vi "MainIdent RT.vi"   [LabVIEW 2018]
doc: "The myRIO Project template acquires acceleration data from the onboard accelerometer and displays the changes of acceleration values in a waveform chart."
uses:
  <vilib>/myRIO/Common/Instrument Driver Framework/myRIO v1.0/Encoder/typedefs/Encoder Signal Mode.ctl
  <vilib>/Platform/TimedLoop/XDataNode/timing_clust.ctl
  <vilib>/Platform/TimedLoop/XDataNode/nitl_modes.ctl
  <vilib>/Platform/TimedLoop/XDataNode/wakeup.ctl
  <vilib>/myRIO/Instrument Drivers/Onboard IO/PWM/typedefs/PWM Reference.ctl
  <vilib>/myRIO/Common/Instrument Driver Framework/Utilities/typedefs/myRIO Generic Hardware Reference.ctl
  <vilib>/myRIO/Common/Instrument Driver Framework/Utilities/typedefs/Hardware Version Enum.ctl
  <vilib>/myRIO/Common/Instrument Driver Framework/Utilities/typedefs/myRIO v1.0 Reference.ctl
  <vilib>/myRIO/Common/Instrument Driver Framework/Utilities/typedefs/Generic FPGA Reference.ctl
  <vilib>/myRIO/Common/Instrument Driver Framework/myRIO v1.0/PWM/typedefs/PWM Channels Enum.ctl
  <vilib>/myRIO/Instrument Drivers/Onboard IO/PWM/typedefs/PWM Configuration.ctl
  <vilib>/userdefined/High Color/nirio_resource_hc.ctl
  <vilib>/myRIO/Common/Instrument Driver Framework/myRIO v1.0/Encoder/typedefs/Encoder Configuration v1.0.ctl
  <vilib>/myRIO/Instrument Drivers/Onboard IO/Encoder/typedefs/Encoder Reference.ctl
  <vilib>/myRIO/Common/Instrument Driver Framework/myRIO v1.0/Encoder/typedefs/Encoder Channels Enum.ctl
  <vilib>/myRIO/Common/Instrument Driver Framework/myRIO v1.0/PWM/vis/myRIO v1.1 Open PWM.vi
  <vilib>/myRIO/Common/Instrument Driver Framework/myRIO v1.0/Encoder/vis/myRIO v1.1 Open Encoder.vi
  <vilib>/myRIO/Common/Instrument Driver Framework/Utilities/vis/Validate Channels.vi
  <vilib>/myRIO/Common/Instrument Driver Framework/myRIO v1.0/PWM/vis/myRIO v1.0 Reserve PWM.vi
  <vilib>/myRIO/Instrument Drivers/Onboard IO/PWM/vis/Set Duty Cycle and Frequency.vi
  <vilib>/myRIO/Common/Instrument Driver Framework/myRIO v1.0/Encoder/vis/myRIO v1.0 Reserve Encoder.vi
  <vilib>/myRIO/Common/Instrument Driver Framework/myRIO v1.0/Encoder/vis/myRIO v1.0 Close Encoder.vi
  <vilib>/myRIO/Common/Instrument Driver Framework/myRIO v1.0/PWM/vis/myRIO v1.0 Close PWM.vi
  <vilib>/myRIO/Common/Instrument Driver Framework/myRIO v1.0/PWM/vis/myRIO v1.0 Build MUX Configuration PWM.vi
  <vilib>/myRIO/Common/Instrument Driver Framework/myRIO v1.0/Resource Manager/vis/myRIO v1.0 Reserve Channel List.vi
  <vilib>/myRIO/Common/Instrument Driver Framework/myRIO v1.0/Encoder/vis/myRIO v1.0 Build MUX Configuration Encoder.vi
  <vilib>/myRIO/Common/Instrument Driver Framework/myRIO v1.0/Encoder/vis/myRIO v1.0 Unreserve Encoder.vi
  <vilib>/myRIO/Common/Instrument Driver Framework/myRIO v1.0/PWM/vis/myRIO v1.0 Unreserve PWM.vi
  <vilib>/myRIO/Common/Instrument Driver Framework/myRIO v1.0/Resource Manager/vis/myRIO v1.0 Create Configuration List.vi
  <vilib>/myRIO/Common/Instrument Driver Framework/myRIO v1.0/Resource Manager/vis/myRIO v1.0 Reserve Channel.vi
  <vilib>/myRIO/Common/Instrument Driver Framework/myRIO v1.0/Resource Manager/vis/myRIO v1.0 Unreserve Channel.vi
  <vilib>/myRIO/Common/Instrument Driver Framework/myRIO v1.0/Resource Manager/vis/myRIO v1.0 Unreserve Channel List.vi
  <vilib>/myRIO/Common/Instrument Driver Framework/myRIO v1.0/Resource Manager/vis/myRIO v1.0 Build Mutex Name.vi
  <vilib>/Utility/VariantDataType/GetNumericInfo.vi
  <vilib>/Utility/error.llb/Error Cluster From Error Code.vi
  <vilib>/myRIO/Common/Instrument Driver Framework/myRIO v1.0/myRIO v1.1 Open.vi
  <vilib>/myRIO/Common/Instrument Driver Framework/Utilities/vis/IO Manager.vi
  <vilib>/myRIO/Common/Instrument Driver Framework/Utilities/vis/Configuration Manager.vi
  <vilib>/myRIO/Common/Instrument Driver Framework/myRIO v1.0/Resource Manager/vis/myRIO v1.0 Configure IO.vi
  <vilib>/myRIO/Common/Instrument Driver Framework/myRIO v1.0/myRIO v1.0 Close.vi
  <vilib>/myRIO/Common/Instrument Driver Framework/myRIO v1.0/PWM/vis/myRIO v1.0 Write PWM.vi
  <vilib>/myRIO/Common/Instrument Driver Framework/myRIO v1.0/Encoder/vis/myRIO v1.0 Configure Encoder.vi
  <vilib>/myRIO/Common/Instrument Driver Framework/myRIO v1.0/Encoder/vis/myRIO v1.0 Enable Encoder.vi
  <vilib>/myRIO/Common/Instrument Driver Framework/myRIO v1.0/Encoder/vis/myRIO v1.0 Read Encoder.vi
  <vilib>/myRIO/Common/Instrument Driver Framework/myRIO v1.0/Encoder/vis/myRIO v1.0 Shutdown Encoder.vi
  <vilib>/myRIO/Common/Instrument Driver Framework/myRIO v1.0/PWM/vis/myRIO v1.0 Shutdown PWM.vi
  <vilib>/platform/TimedLoop/XDataNode/XDataNode.xnode
  <vilib>/myRIO/Instrument Drivers/Onboard IO/PWM/vis/myRIO PWM Open.xnode
  <vilib>/myRIO/Instrument Drivers/Onboard IO/Encoder/vis/myRIO Encoder Open.xnode
  <vilib>/Platform/TimedLoop/XDataNode/XDNodeRunTimeDep.lvlib
  <vilib>/myRIO/Instrument Drivers/Onboard IO/Encoder/Encoder.lvlib
  <vilib>/myRIO/Instrument Drivers/Onboard IO/PWM/PWM.lvlib
types:
  T1 = typedef "Encoder Signal Mode.ctl" = enum16{"Quadrature phase signal", "Step and direction signal"}
  T2 = typedef "PWM.lvlib/PWM Reference.ctl" = cluster{"myRIO Reference":T3, "PWM Channels Enum":T7, "PWM Configuration":T8}
  T3 = typedef "myRIO Generic Hardware Reference.ctl" = cluster{"myRIO Model":T4, "myRIO Hardware Reference":T5}
  T4 = typedef "Hardware Version Enum.ctl" = enum16{"Unknown", "myRIO-1900", "myRIO-1950", "roboRIO", "NI ELVIS RIO CM", "ELVIS III"}
  T5 = typedef "myRIO v1.0 Reference.ctl" = cluster{"Generic FPGA Reference":T6, "Allow multiple opens":bool}
  T6 = typedef "Generic FPGA Reference.ctl" = refnum<k20>
  T7 = typedef "PWM Channels Enum.ctl" = enum16{"Not Connected", "C/PWM0", "C/PWM1", "A/PWM0", "A/PWM1", "A/PWM2", "A/PWM3", "A/PWM4", "A/PWM5", "A/PWM6", "A/PWM7", "A/PWM8", "A/PWM9", "A/PWM10", "A/PWM11", "A/PWM12", "A/PWM13", "A/PWM14", "A/PWM15", "A/PWM16", "A/PWM17", "A/PWM18", "A/PWM19", "B/PWM0", "B/PWM1", "B/PWM2", "B/PWM3", "B/PWM4", "B/PWM5", "B/PWM6", "B/PWM7", "B/PWM8", "B/PWM9", "B/PWM10", "B/PWM11", "B/PWM12", "B/PWM13", "B/PWM14", "B/PWM15", "B/PWM16", "B/PWM17", "B/PWM18", "B/PWM19", "PWM/PWM0", "PWM/PWM1", "PWM/PWM2", "PWM/PWM3", "PWM/PWM4", "PWM/PWM5", "PWM/PWM6", "PWM/PWM7", "PWM/PWM8", "PWM/PWM9"}
  T8 = typedef "PWM.lvlib/PWM Configuration.ctl" = cluster{"Frequency":dbl, "Duty Cycle":dbl}
  T9 = typedef "Encoder.lvlib/Encoder Reference.ctl" = cluster{"myRIO Reference":T3, "Encoder Channels Enum":T10}
  T10 = typedef "Encoder Channels Enum.ctl" = enum16{"Not Connected", "C/ENC0", "C/ENC1", "A/ENC", "A/ENC0", "A/ENC1", "A/ENC2", "A/ENC3", "A/ENC4", "A/ENC5", "A/ENC6", "A/ENC7", "A/ENC8", "A/ENC9", "B/ENC", "B/ENC0", "B/ENC1", "B/ENC2", "B/ENC3", "B/ENC4", "B/ENC5", "B/ENC6", "B/ENC7", "B/ENC8", "B/ENC9", "DIO/ENC0", "DIO/ENC1", "DIO/ENC2", "DIO/ENC3", "DIO/ENC4"}
  T11 = typedef "XDNodeRunTimeDep.lvlib/timing_clust.ctl" = cluster{"Expected End [f-1]":u64, "Actual End [f-1]":u64, "Finished Late? [f-1]":bool, "Expected End [i-1]":u64, "Actual End [i-1]":u64, "Finished Late? [i-1]":bool, "Expected Start [i]":u64, "Actual Start [i]":u64, "Expected Start [f]":u64, "Actual Start [f]":u64, "Source Name":string, "Structure Name":string, "Period":i64, "Deadline":i64, "Offset":i64, "Start":i64, "Priority":i32, "Timeout":i32, "Mode":T12, "Wakeup Reason":T13, "Error":errorcluster, "Source Type":string, "Secondary Source Type":string, "Global End Time":u64, "Global Start Time":u64, "Frame Duration":u64, "Iteration Duration":u64, "Assigned CPU":i32, "I/O Scan Engine Mode":u32}
  T12 = typedef "XDNodeRunTimeDep.lvlib/nitl_modes.ctl" = enum32{"No Change", "Process missed periods, maintain original phase", "Discard missed periods, maintain original phase", "Process missed periods, ignore original phase", "Discard missed periods, ignore original phase"}
  T13 = typedef "XDNodeRunTimeDep.lvlib/wakeup.ctl" = enum32{"Normal", "Aborted", "Asynchronous wakeup", "Timing source error", "Timed loop error", "Timeout"}
  T14 = cluster{"Double":dbl, dbl, dbl, "seconds since 1Jan1904":timestamp}
  T15 = cluster{"Double":dbl, "dbl Scaled Value":dbl, "Output":dbl, "seconds since 1Jan1904":timestamp}
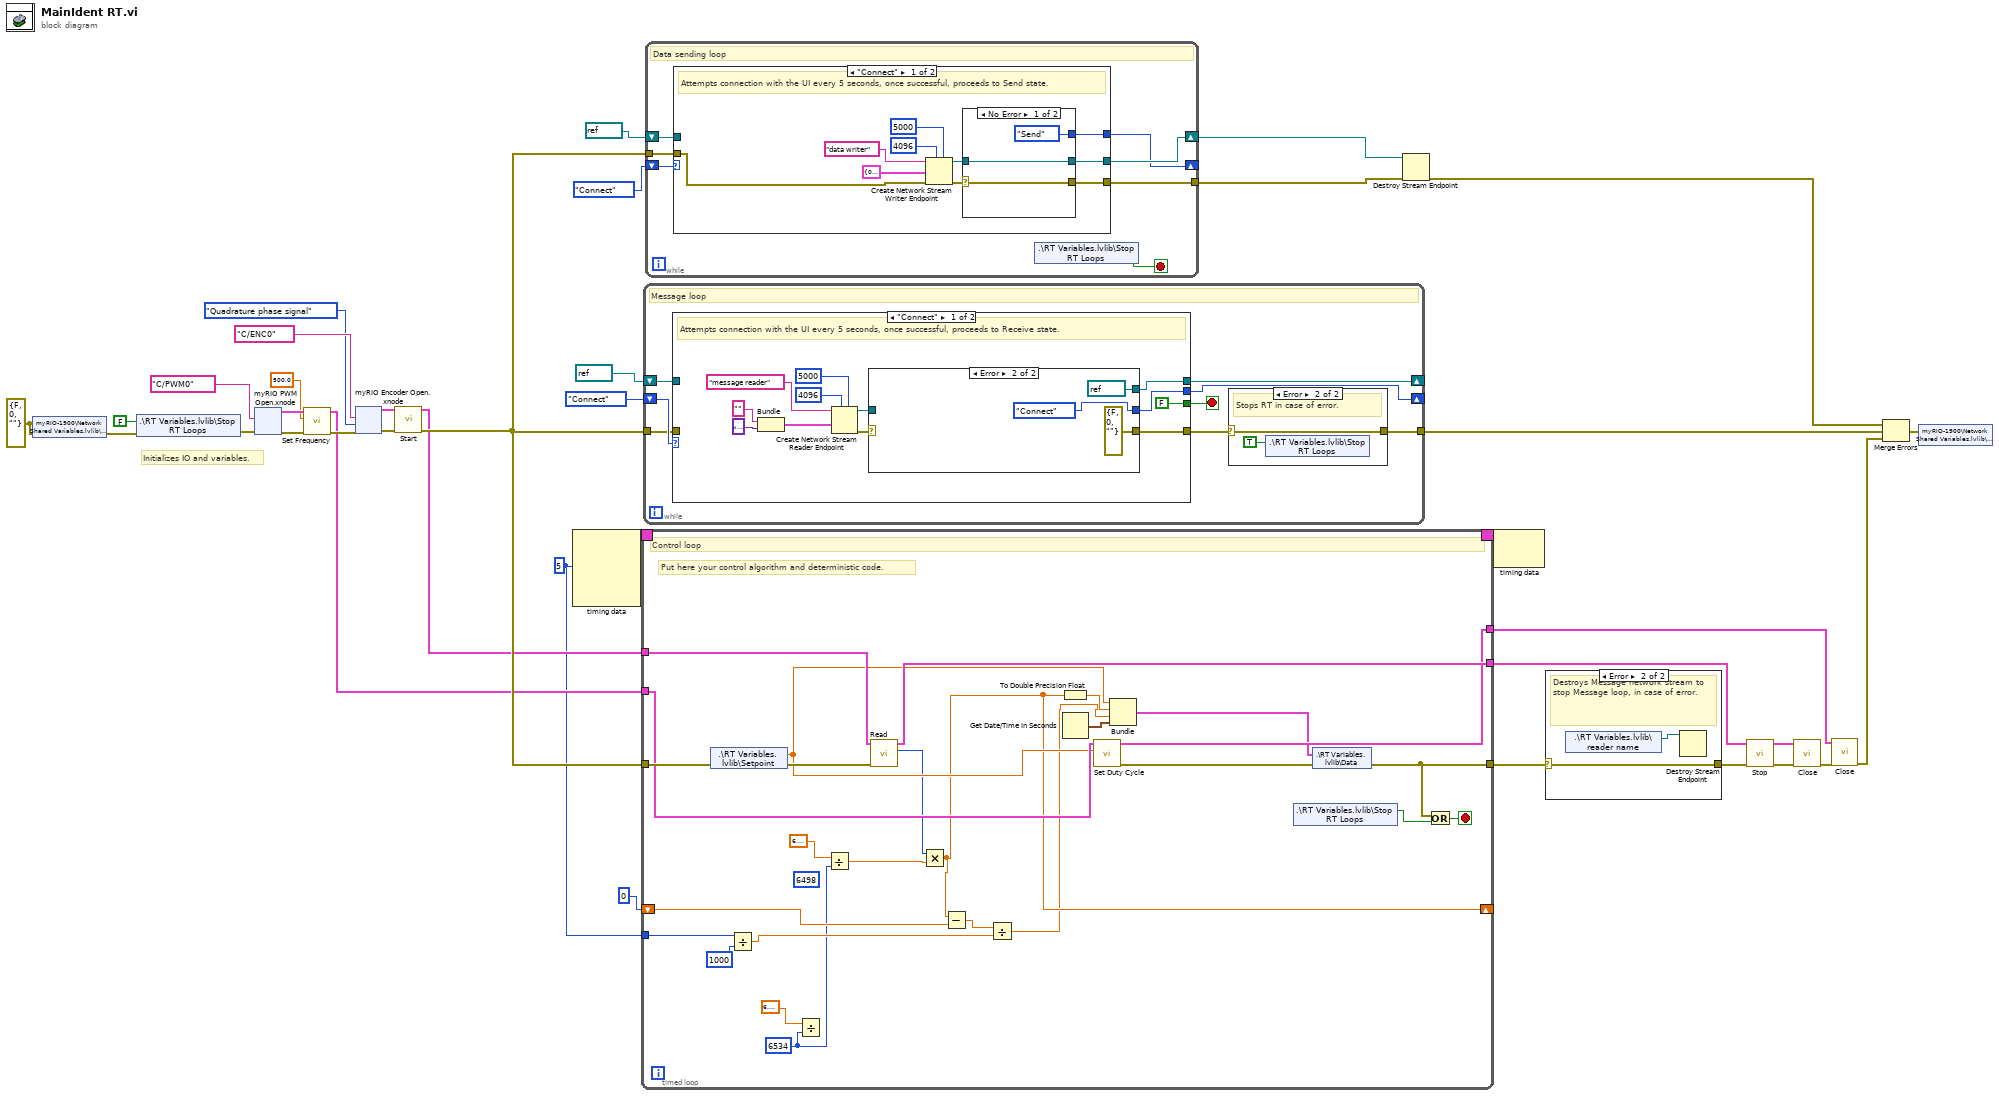
[diagram p0: block diagram]
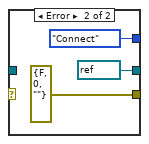
[diagram p3: hidden frame]
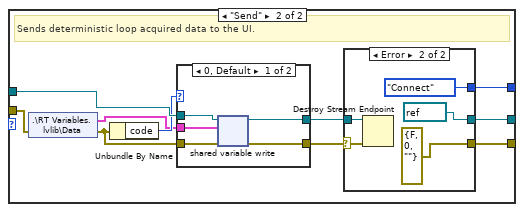
[diagram p4: hidden frame]
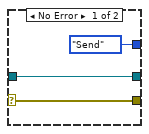
[diagram p5: hidden frame]
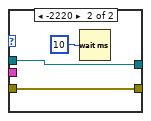
[diagram p6: hidden frame]
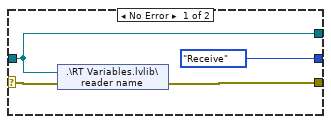
[diagram p8: hidden frame]
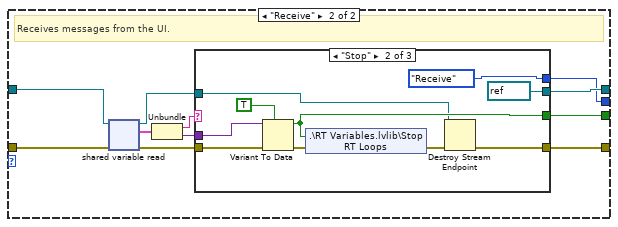
[diagram p9: hidden frame]
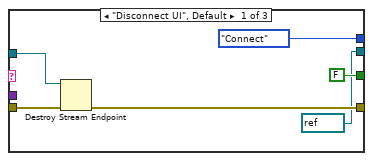
[diagram p10: hidden frame]
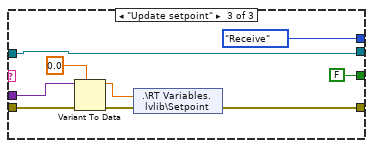
[diagram p11: hidden frame]
diagram:
  w1 = i64 5 ("Period")
  w24 = errorcluster {"status"=FALSE, "code"=0, "source"=""} ("error IO")
  # "Initializes IO and variables."
  n1 = shared-variable "myRIO-1900\\Network Shared Variables.lvlib\\error IO"(w24, error in=w24) -> (error out=w25:errorcluster)
  n2 = shared-variable ".\\RT Variables.lvlib\\Stop RT Loops"(FALSE ("Stop RT Loops"), error in=w25) -> (error out=w10:errorcluster)
  n3 = xnode "myRIO PWM Open.xnode"("error in (no error)"=w10, "Channel Name"=tag "C/PWM0") -> ("error out"=w12:errorcluster, "PWM Ref Out"=w11:T2)  [unwired: 1 in]
  n4 = call <vilib>:"Set Frequency.vi"("error in (no error)"=w12, "Frequency [Hz]"=500.0, "PWM Ref In"=w11) -> ("error out"=w9:errorcluster, "PWM Ref Out"=w6:T2)  [unwired: 6 in]
  n5 = xnode "myRIO Encoder Open.xnode"("error in (no error)"=w9, "Channel Name"=tag "C/ENC0", "Encoder Signal Mode"=Encoder_Signal_Mode."Quadrature phase signal") -> ("error out"=w21:errorcluster, "Encoder Ref Out"=w20:T9)  [unwired: 2 in]
  n6 = call <vilib>:"Start.vi"("error in (no error)"=w21, "Encoder Ref In"=w20) -> ("error out"=w18:errorcluster, "Encoder Ref Out"=w17:T9)  [unwired: 8 in]
  n7 = node-c288(w1) -> (w37:T11)  [unwired: 3 in]
  n8 = timed-loop {
    timing: w37 -> [_]
    timing-out: [_] -> w36
    tunnel: w18 -> [w62]
    tunnel: [w58] -> w23
    tunnel: w17 -> [w57]
    tunnel: [w56] -> w13
    tunnel: w6 -> [w54]
    tunnel: [w52] -> w5
    shift-right: [w45] -> _
    shift-left: 0 -> [w44]
    tunnel: w1 -> [w41]
    stop <- w59 stop-if-true
    w38 = 6534
    (unwired) 6498
    # "Put here your control algorithm and deterministic code."
    # "Control loop"
    n9 = shared-variable ".\\RT Variables.lvlib\\Setpoint"(error in=w62) -> (w50:dbl, error out=w63:errorcluster)
    n10 = Divide(x=w41, y=1000) -> (x/y=w39:dbl)
    n11 = Divide(x=6.283185307179586, y=w38) -> ()  [unwired: 1 out]
    n12 = Divide(x=6.283185307179586, y=w38) -> (x/y=w46:dbl)
    n13 = call <vilib>:"Read.vi"("error in (no error)"=w63, "Encoder Ref In"=w57) -> ("Counter Value"=w47:i32, "Encoder Ref Out"=w56:T9)  [unwired: 5 in, 3 out]
    n14 = Multiply(x=w47, y=w46) -> (x*y=w45:dbl)
    n15 = Subtract(x=w45, y=w44) -> (x-y=w43:dbl)
    n16 = Divide(x=w43, y=w39) -> (x/y=w42:dbl)
    n17 = To Double Precision Float(number=w45) -> (double precision float=w53:dbl)
    n18 = Get Date/Time In Seconds() -> (seconds since 1Jan1904=w61:timestamp)
    n19 = call <vilib>:"Set Duty Cycle.vi"("Duty Cycle"=w50, "PWM Ref In"=w54) -> ("error out"=w55:errorcluster, "PWM Ref Out"=w52:T2)  [unwired: 7 in]
    n20 = Bundle("Double"=w50, w53, w42, "seconds since 1Jan1904"=w61) -> (w51:T14)  [unwired: 1 in]
    n21 = shared-variable ".\\RT Variables.lvlib\\Stop RT Loops"() -> (w60:bool)  [unwired: 1 in, 1 out]
    n22 = shared-variable ".\\RT Variables.lvlib\\Data"(w51, error in=w55) -> (error out=w58:errorcluster)
    n23 = Or(x=w58, y=w60) -> (x .or. y?=w59:bool)
  }
  n24 = while {
    tunnel: [w66] -> w27
    shift-right: [w72] -> _
    shift-left: refnum<k21> refnum ("reader name") -> [w70]
    shift-right: [w71] -> _
    shift-left: enum16{"Connect", "Receive"}."Connect" ("Message states") -> [w73]
    tunnel: w18 -> [w68]
    stop <- w69 stop-if-true
    # "Message loop"
    n25 = case shown="\"Connect\"" w73 {
      tunnel: [w79 w99] -> w67
      tunnel: [w78 w101] -> w72
      tunnel: [w86 w96] -> w71
      tunnel: w70 -> [_ w106]
      tunnel: w68 -> [_ w98]
      tunnel: [FALSE ("Stop RT Loops") w97] -> w69
      frame "Connect" {
        # "Attempts connection with the UI every 5 seconds, once successful, proceeds to Receive state."
        n26 = Bundle("", variant) -> (w82:cluster{string, variant})  [unwired: 1 in]
        n27 = Create Network Stream Reader Endpoint(5:5000 ("timeout in ms (-1)"), 7:4096 ("reader buffer size"), 9:w82, 11:"message reader" ("reader name")) -> (0:w81:errorcluster, 3:w77:refnum<k21>)  [unwired: 3 in]
        n28 = case shown="Error" w81 {
          selector: w81 -> [w90 _]
          tunnel: [enum16{"Connect", "Receive"}."Receive" ("Message states") enum16{"Connect", "Receive"}."Connect" ("Message states")] -> w86
          tunnel: [w89 errorcluster {"status"=FALSE, "code"=0, "source"=""} ("error IO")] -> w79
          tunnel: [w91 refnum<k21> refnum ("reader name")] -> w78
          tunnel: w77 -> [w91 _]
          frame No Error {
            n29 = shared-variable ".\\RT Variables.lvlib\\reader name"(w91, error in=w90) -> (error out=w89:errorcluster)
          }
          frame Error {
          }
        }
      }
      frame "Receive" {
        # "Receives messages from the UI."
        n30 = shared-variable-read(w106, w98) -> (w100:refnum<k21>, w102:errorcluster, w105:cluster{string, variant})  [unwired: 1 in, 1 out]
        n31 = Unbundle(w105) -> (w104:string, w103:variant)
        n32 = case shown="\"Stop\"" w104 {
          tunnel: w103 -> [_ w120 w131]
          tunnel: w102 -> [w110 w122 w130]
          tunnel: [w109 w116 w126] -> w99
          tunnel: [refnum<k21> refnum ("reader name") refnum<k21> refnum ("reader name") w125] -> w101
          tunnel: w100 -> [w108 w115 w125]
          tunnel: [FALSE ("Stop RT Loops") w119 FALSE ("Stop RT Loops")] -> w97
          tunnel: [enum16{"Connect", "Receive"}."Connect" ("Message states") enum16{"Connect", "Receive"}."Receive" ("Message states") enum16{"Connect", "Receive"}."Receive" ("Message states")] -> w96
          frame "Disconnect UI", Default {
            n33 = Destroy Stream Endpoint(8:w110, 11:w108) -> (0:w109:errorcluster)
          }
          frame "Stop" {
            n34 = Variant To Data(error in=w122, type=TRUE ("Stop RT Loops"), Variant=w120) -> (data=w119:bool, error out=w121:errorcluster)
            n35 = shared-variable ".\\RT Variables.lvlib\\Stop RT Loops"(w119, error in=w121) -> (error out=w117:errorcluster)
            n36 = Destroy Stream Endpoint(8:w117, 11:w115) -> (0:w116:errorcluster)
          }
          frame "Update setpoint" {
            n37 = Variant To Data(error in=w130, type=0.0, Variant=w131) -> (data=w128:dbl, error out=w127:errorcluster)
            n38 = shared-variable ".\\RT Variables.lvlib\\Setpoint"(w128, error in=w127) -> (error out=w126:errorcluster)
          }
        }
      }
    }
    n39 = case shown="Error" w67 {
      selector: w67 -> [w74 w75]
      tunnel: [w74 w75] -> w66
      frame No Error {
        # "No action required."
      }
      frame Error {
        # "Stops RT in case of error."
        n40 = shared-variable ".\\RT Variables.lvlib\\Stop RT Loops"(TRUE ("Stop RT Loops")) -> ()  [unwired: 1 in, 1 out]
      }
    }
  }
  n41 = while {
    shift-right: [w136] -> w30
    shift-left: refnum<k21> refnum ("writer endpoint") -> [w134]
    tunnel: [w135] -> w31
    tunnel: w18 -> [w133]
    shift-right: [w132] -> _
    shift-left: enum16{"Connect", "Send"}."Connect" ("Message states") -> [w137]
    stop <- w138 stop-if-true
    # "Data sending loop"
    n42 = case shown="\"Connect\"" w137 {
      tunnel: [w141 w157] -> w135
      tunnel: [w139 w155] -> w136
      tunnel: [w146 w158] -> w132
      tunnel: w134 -> [_ w164]
      tunnel: w133 -> [w142 w163]
      frame "Connect" {
        # "Attempts connection with the UI every 5 seconds, once successful, proceeds to Send state."
        n43 = Create Network Stream Writer Endpoint(5:5000 ("timeout in ms (-1)"), 7:4096 ("writer buffer size"), 8:w142, 9:T15 {"Double"=0.0, "dbl Scaled Value"=0.0, "Output"=0.0, "seconds since 1Jan1904"=timestamp(0 s since 1904-01-01)} ("Data"), 11:"data writer" ("writer name")) -> (0:w144:errorcluster, 3:w140:refnum<k21>)  [unwired: 2 in]
        n44 = case shown="No Error" w144 {
          selector: w144 -> [w149 _]
          tunnel: [enum16{"Connect", "Send"}."Send" ("Message states") enum16{"Connect", "Send"}."Connect" ("Message states")] -> w146
          tunnel: [w149 errorcluster {"status"=FALSE, "code"=0, "source"=""} ("error IO")] -> w141
          tunnel: w140 -> [w151 _]
          tunnel: [w151 refnum<k21> refnum ("writer endpoint")] -> w139
          frame No Error {
          }
          frame Error {
          }
        }
      }
      frame "Send" {
        # "Sends deterministic loop acquired data to the UI."
        n45 = shared-variable ".\\RT Variables.lvlib\\Data"(error in=w163) -> (w160:T15, error out=w162:errorcluster)
        n46 = Unbundle By Name(w162) -> ("code"=w161:i32)
        n47 = case shown="0, Default" w161 {
          tunnel: [w177 w179] -> w159
          tunnel: [w176 w178] -> w156
          tunnel: w164 -> [w175 w178]
          tunnel: w162 -> [w174 w179]
          tunnel: w160 -> [w173 _]
          frame 0, Default {
            n48 = shared-variable-write(w175, w174, w173) -> (w176:refnum<k21>, w177:errorcluster)  [unwired: 1 in, 1 out]
          }
          frame -2220 {
            n49 = Wait (ms)(milliseconds to wait=u32 10) -> ()  [unwired: 1 out]
          }
        }
        n50 = case shown="Error" w159 {
          selector: w159 -> [w167 w171]
          tunnel: [enum16{"Connect", "Send"}."Send" ("Message states") enum16{"Connect", "Send"}."Connect" ("Message states")] -> w158
          tunnel: [w167 errorcluster {"status"=FALSE, "code"=0, "source"=""} ("error IO")] -> w157
          tunnel: w156 -> [w165 w170]
          tunnel: [w165 refnum<k21> refnum ("writer endpoint")] -> w155
          frame No Error {
          }
          frame Error {
            n51 = Destroy Stream Endpoint(8:w171, 11:w170) -> ()  [unwired: 1 out]
          }
        }
      }
    }
    n52 = shared-variable ".\\RT Variables.lvlib\\Stop RT Loops"() -> (w138:bool)  [unwired: 1 in, 1 out]
  }
  n53 = Destroy Stream Endpoint(8:w31, 11:w30) -> (0:w28:errorcluster)
  n54 = node-c288(w36) -> ()  [unwired: 1 out]
  n55 = case shown="Error" w23 {
    selector: w23 -> [w181 w182]
    tunnel: [w181 w182] -> w14
    frame No Error {
      # "No action required."
    }
    frame Error {
      # "Destroys Message network stream to stop Message loop, in case of error."
      n56 = shared-variable ".\\RT Variables.lvlib\\reader name"() -> (w183:refnum<k21>)  [unwired: 1 in, 1 out]
      n57 = Destroy Stream Endpoint(11:w183) -> ()  [unwired: 1 in, 1 out]
    }
  }
  n58 = call <vilib>:"Stop.vi"("error in (no error)"=w14, "Encoder Ref In"=w13) -> ("error out"=w15:errorcluster, "Encoder Ref Out"=w16:T9)  [unwired: 8 in]
  n59 = call <vilib>:"Close.vi"("error in (no error)"=w15, "Encoder Ref In"=w16) -> ("error out"=w8:errorcluster)  [unwired: 9 in]
  n60 = call <vilib>:"Close.vi"("error in (no error)"=w8, "PWM Ref In"=w5) -> ("error out"=w7:errorcluster)  [unwired: 9 in]
  n61 = Merge Errors(w28, w27, w7) -> (w26:errorcluster)
  n62 = shared-variable "myRIO-1900\\Network Shared Variables.lvlib\\error IO"(w26) -> ()  [unwired: 1 in, 1 out]
